vi "mod_Downconvert extracted signals.vi"(0 "extracted AM modulated wfm (IF)":waveform(dbl), 2 "carrier frequency":dbl, 5 "extracted pilot tone wfm (IF)":waveform(dbl), 7 "passband bandwidth (AM modulated wfm)":dbl, 9 "passband bandwidth (pilot tone wfm)":dbl, 11 "error in (no error)":errorcluster, 13 "reset? (T)":bool=TRUE) -> (4 "extracted AM modulated signal (baseband)":cluster{"t0":dbl, "dt":dbl, "Y":cdb[]}={"t0"=0.0, "dt"=1.0, "Y"=[]} {"Y" format="%.3f"; "dt" format="%^.2e"; "t0" format="%.4f"}, 6 "extracted pilot tone (baseband)":cluster{"t0":dbl, "dt":dbl, "Y":cdb[]}={"t0"=0.0, "dt"=1.0, "Y"=[]} {"Y" format="%.3f"; "dt" format="%^.2e"; "t0" format="%.4f"}, 8 "downconversion filter length":i32, 15 "error out":errorcluster)   [LabVIEW 2020, in "niAMT.lvlib"]
uses:
  <vilib>/addons/Modulation/niAMT.lvlib
  <vilib>/addons/Modulation/Analog/MT Downconvert Passband (Real).vi
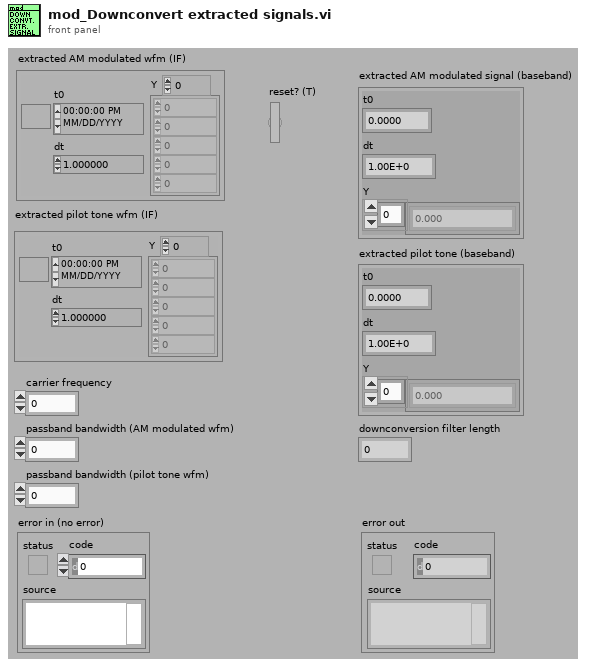
[diagram p1: front panel]
types:
  T1 = typedef "niAMT.lvlib/Complex Data Waveform.ctl" = cluster{"t0":dbl, "dt":dbl, "Y":cdb[]}
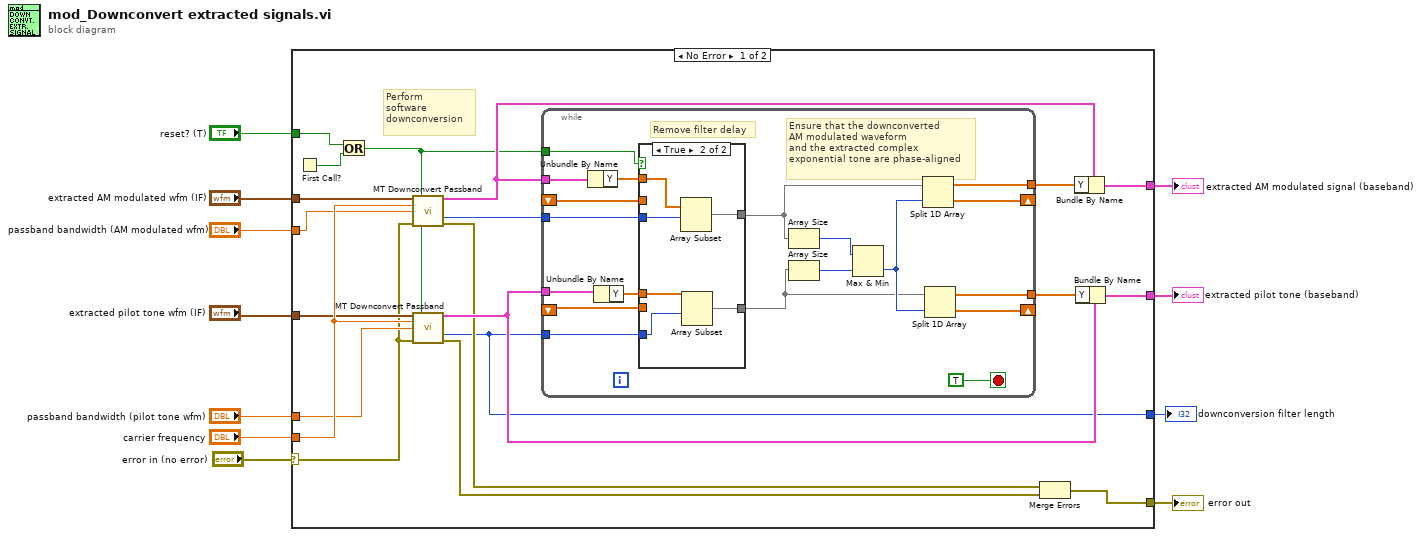
[diagram p0: block diagram]
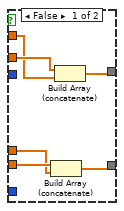
[diagram p2: hidden frame]
diagram:
  n1 = case shown="No Error" "error in (no error)" {
    selector: "error in (no error)" -> [w18 w63]
    tunnel: "extracted AM modulated wfm (IF)" -> [w31 _]
    tunnel: "carrier frequency" -> [w30 _]
    tunnel: "passband bandwidth (AM modulated wfm)" -> [w29 _]
    tunnel: "passband bandwidth (pilot tone wfm)" -> [w28 _]
    tunnel: "reset? (T)" -> [w21 _]
    tunnel: [w26 _] -> w7
    tunnel: [w23 _] -> w6
    tunnel: "extracted pilot tone wfm (IF)" -> [w22 _]
    tunnel: [w15 w63] -> w2
    tunnel: [w12 _] -> w1
    frame No Error {
      # "Perform\nsoftware\ndownconversion"
      n2 = First Call?() -> (First Call?: T/F=w20:bool)
      n3 = Or(x=w21, y=w20) -> (x .or. y?=w19:bool)
      n4 = call-poly <vilib>:"MT Downconvert Passband.vi"("Waveform"=w31, "reset? (F)"=w19, "carrier frequency (Hz)"=w30, "passband bandwidth (Hz)"=w29, "error in (no error)"=w18) -> ("downconverted waveform (complex baseband)"=w27:T1, "filter length"=w13:i32, "error out"=w17:errorcluster)  [unwired: 2 in, 6 out]
      n5 = call-poly <vilib>:"MT Downconvert Passband.vi"("Waveform"=w22, "reset? (F)"=w19, "carrier frequency (Hz)"=w30, "passband bandwidth (Hz)"=w28, "error in (no error)"=w18) -> ("downconverted waveform (complex baseband)"=w25:T1, "filter length"=w12:i32, "error out"=w16:errorcluster)  [unwired: 2 in, 6 out]
      n6 = while {
        tunnel: w19 -> [w50]
        tunnel: w27 -> [w49]
        tunnel: w25 -> [w48]
        tunnel: w13 -> [w45]
        tunnel: w12 -> [w44]
        shift-right: [w38] -> _
        shift-left: _ -> [w36]
        shift-right: [w37] -> _
        shift-left: _ -> [w35]
        tunnel: [w34] -> w14
        tunnel: [w33] -> w24
        stop <- TRUE stop-if-true
        # "Ensure that the downconverted\nAM modulated waveform\nand the extracted complex\nexponential tone are phase-aligned"
        # "Remove filter delay"
        n7 = Unbundle By Name(w49) -> ("Y"=w47:cdb[])
        n8 = Unbundle By Name(w48) -> ("Y"=w46:cdb[])
        n9 = case shown="True" w50 {
          tunnel: w47 -> [w55 w62]
          tunnel: w46 -> [w52 w61]
          tunnel: w45 -> [_ w58]
          tunnel: w44 -> [_ w57]
          tunnel: [w54 w60] -> w41
          tunnel: [w51 w59] -> w39
          tunnel: w36 -> [w56 _]
          tunnel: w35 -> [w53 _]
          frame False {
            n10 = Build Array (concatenate)(w53, w52) -> (w51:cdb[])
            n11 = Build Array (concatenate)(w56, w55) -> (w54:cdb[])
          }
          frame True {
            n12 = Array Subset(array=w62, index=w58) -> (w60:cdb[])  [unwired: 1 in]
            n13 = Array Subset(array=w61, index=w57) -> (w59:cdb[])  [unwired: 1 in]
          }
        }
        n14 = Array Size(array=w41) -> (size(s)=w43:i32)
        n15 = Array Size(array=w39) -> (size(s)=w42:i32)
        n16 = Max & Min(x=w43, y=w42) -> (min(x,y)=w40:i32)  [unwired: 1 out]
        n17 = Split 1D Array(array=w41, index=w40) -> (first subarray=w34:cdb[], second subarray=w38:cdb[])
        n18 = Split 1D Array(array=w39, index=w40) -> (first subarray=w33:cdb[], second subarray=w37:cdb[])
      }
      n19 = Merge Errors(w17, w16) -> (w15:errorcluster)
      n20 = Bundle By Name(cluster=w27, "Y"=w14) -> (w26:T1)
      n21 = Bundle By Name(cluster=w25, "Y"=w24) -> (w23:T1)
    }
    frame Error {
    }
  }
  "extracted AM modulated signal (baseband)" <- w7
  "extracted pilot tone (baseband)" <- w6
  "error out" <- w2
  "downconversion filter length" <- w1
